vi "Get Cursor Position.vi"(8 "error in (no error)":errorcluster) -> (0 "error out":errorcluster, 2 "Y":i32, 3 "X":i32)   [LabVIEW 2020, in "MacroAssert.lvlib"]
uses:
  MacroAssert.lvlib
  user32.dll
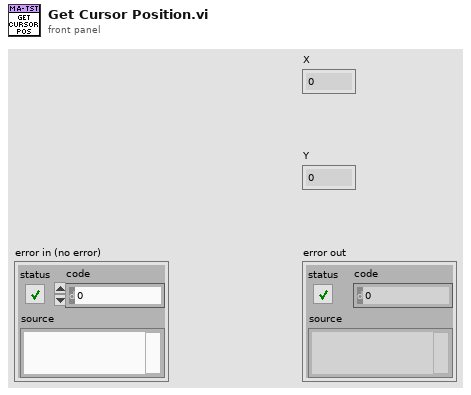
[diagram p1: front panel]
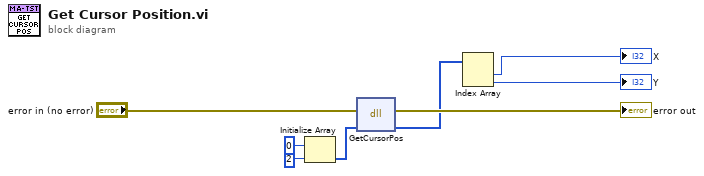
[diagram p0: block diagram]
diagram:
  n1 = Initialize Array(0, 2) -> (w6:i32[])
  n2 = dll-call lib="USER32.DLL" fn="GetCursorPos"(error in="error in (no error)", "POINT"=w6) -> (error out=→"error out":errorcluster, "POINT"=w3:i32[])  [unwired: 2 in, 2 out]
  n3 = Index Array(array=w3) -> (element #1=→"X":i32, element #2=→"Y":i32)  [unwired: 2 in]
